vi "Lvi Strain Channel Settings.vi"(0 "TaskRef":i32, 1 "Channel":u32, 2 "BridgeType":i32, 3 "BridgeExcitationSource":i32, 4 "ExcitationVoltage":dbl, 5 "GageResistance":dbl, 6 "GageFactor":dbl, 7 "error in (no error)":errorcluster, 8 "WireResistance":dbl, 9 "PoissonRatio":dbl, 10 "UnstrainedVoltage":dbl, 11 "ShuntCorrection":dbl) -> (20 "TaskRef out":i32, 21 "function return":i32, 27 "error out":errorcluster)   [LabVIEW 2022 SP3, in "DtLvLink.lvlib"]
doc: "Calls directly into the entry points of the DLL of the Data Acq SDK to set the properties of a strain gage sensor."
uses:
  DtLvLink.lvlib
  <userlib>/LV-Link3/DtLvLink_64.dll
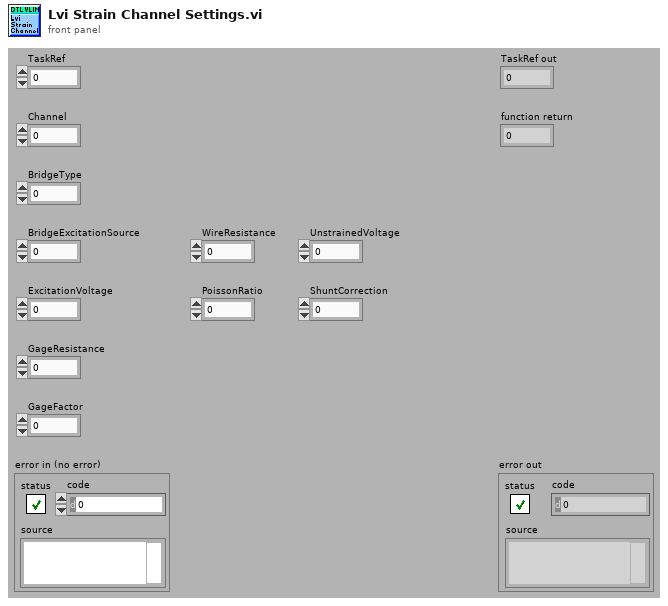
[diagram p1: front panel]
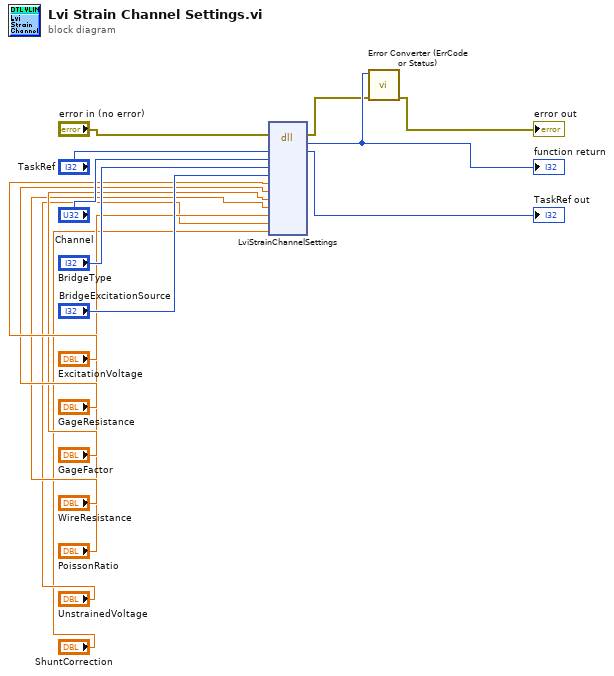
[diagram p0: block diagram]
diagram:
  n1 = dll-call lib="C:/Program Files/National Instruments/LabVIEW 2022/user.lib/LV-Link3/DtLvLink_64.*" fn="LviStrainChannelSettings"(error in="error in (no error)", "TaskRef"="TaskRef", "Channel"="Channel", "BridgeType"="BridgeType", "BridgeExcitationSource"="BridgeExcitationSource", "ExcitationVoltage"="ExcitationVoltage", "GageResistance"="GageResistance", "GageFactor"="GageFactor", "WireResistance"="WireResistance", "PoissonRatio"="PoissonRatio", "UnstrainedVoltage"="UnstrainedVoltage", "ShuntCorrection"="ShuntCorrection") -> (error out=w2:errorcluster, "return type"=w16:i32, "TaskRef"=→"TaskRef out":i32)  [unwired: 12 in, 1 out]
  "function return" <- w16
  n2 = call "Error Converter (ErrCode or Status).vi"("error in (no error)"=w2, "error code"=w16) -> ("error out"=→"error out":errorcluster)  [unwired: 9 in]
